vi "aula 2.vi"() -> ()   [LabVIEW 2026]
panel:
  in  "Boolean":bool
  in  "stop":bool
  out "Numeric":i32
  out "x*y":dbl
  out "°C":dbl(slide) scale=0.0..300.0
  in  "°F":dbl(slide) scale=0.0..300.0
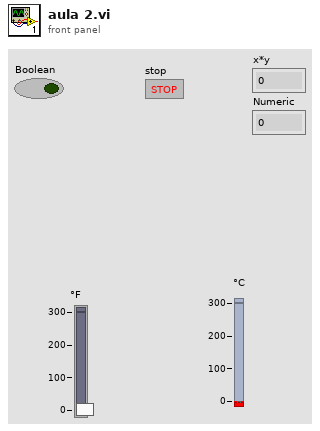
[diagram p1: front panel]
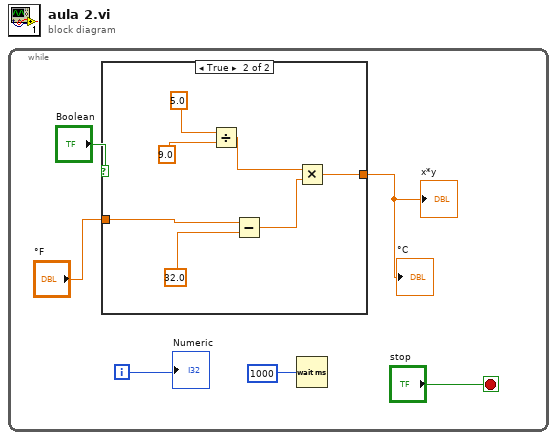
[diagram p0: block diagram]
diagram:
  n1 = while {
    i -> [w5]
    stop <- "stop" stop-if-true
    n2 = case shown="True" "Boolean" {
      tunnel: [w7 w9] -> w6
      tunnel: "°F" -> [w7 w8]
      frame False {
      }
      frame True {
        n3 = Divide(x=5.0, y=9.0) -> (x/y=w12:dbl)
        n4 = Subtract(x=w8, y=32.0) -> (x-y=w13:dbl)
        n5 = Multiply(x=w12, y=w13) -> (x*y=w9:dbl)
      }
    }
    "°C" <- w6
    "x*y" <- w6
    n6 = Wait (ms)(milliseconds to wait=u32 1000) -> ()  [unwired: 1 out]
    "Numeric" <- w5
  }
